vi "Match Type.vi"(7 "raise for mismatch?":bool, 8 "error in (no error)":errorcluster, 10 "type code":T1, 11 "NT Scalar (Numeric) in":refnum<class "NT Scalar (Numeric).lvclass">) -> (0 "error out":errorcluster, 1 "type match?":bool, 2 "type code out":T1, 3 "NT Scalar (Numeric) out":refnum<class "NT Scalar (Numeric).lvclass">)   [LabVIEW 2020, in "PV Access.lvlib" / "PV Data.lvlib" / "NT Scalar (Numeric).lvclass"]
uses:
  NT Scalar (Numeric).lvclass
  <vilib>/ErrorRing/Error Ring.xnode
  PV Data.lvlib
  <vilib>/Utility/error.llb/Error Cluster From Error Code.vi
  Type Code.ctl
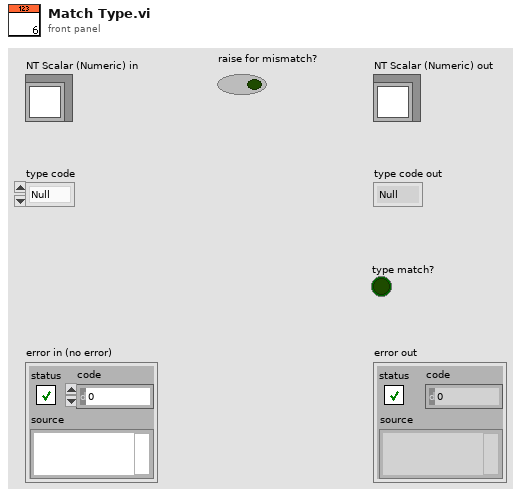
[diagram p1: front panel]
types:
  T1 = typedef "PV Access.lvlib/PV Data.lvlib/Type Code.ctl" = enum8{"Null", "Bool", "BoolA", "Int8", "Int8A", "Int16", "Int16A", "Int32", "Int32A", "Int64", "Int64A", "UInt8", "UInt8A", "UInt16", "UInt16A", "UInt32", "UInt32A", "UInt64", "UInt64A", "Float32", "Float32A", "Float64", "Float64A", "String", "StringA", "Struct", "StructA", "Union", "UnionA", "Any", "AnyA"}
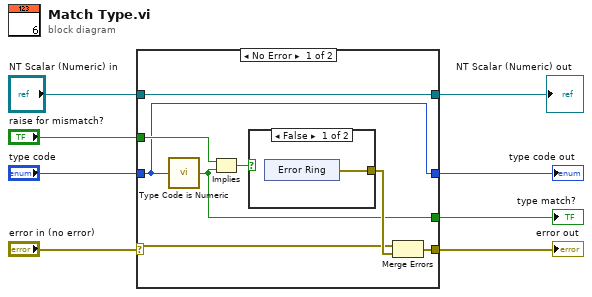
[diagram p0: block diagram]
diagram:
  n1 = case shown="No Error" "error in (no error)" {
    selector: "error in (no error)" -> [w12 w24]
    tunnel: [w11 w24] -> w3
    tunnel: [w16 w23] -> w6
    tunnel: "NT Scalar (Numeric) in" -> [w16 w23]
    tunnel: "type code" -> [w10 w22]
    tunnel: [w9 _] -> w2
    tunnel: "raise for mismatch?" -> [w15 _]
    tunnel: [w10 w22] -> w1
    frame No Error {
      n2 = call "Type Code is Numeric.vi"("type code"=w10) -> ("is match?"=w9:bool)
      n3 = Implies(1:w9, 2:w15) -> (0:w14:bool)
      n4 = case shown="False" w14 {
        tunnel: [w17 _] -> w13
        frame False {
          n5 = xnode "Error Ring"() -> ("error out"=w17:errorcluster)
        }
        frame True {
        }
      }
      n6 = Merge Errors(w12, w13) -> (w11:errorcluster)
    }
    frame Error {
    }
  }
  "error out" <- w3
  "type match?" <- w2
  "NT Scalar (Numeric) out" <- w6
  "type code out" <- w1
